vi "Slog1.vi"(2 "z":dbl[](array[numeric]), 3 "T":dbl[](array[numeric])) -> (0 "dY":dbl[](array[numeric]), 1 "Y":dbl[](array[numeric]))   [LabVIEW 2022 SP3]
uses:
  <vilib>/express/express arith-compare/Formula/XNode/ExpressFormulaBlockNode.xnode
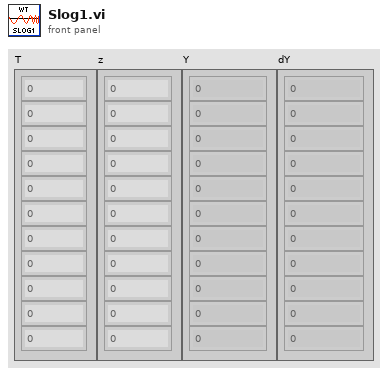
[diagram p1: front panel]
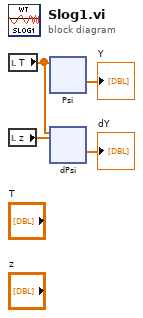
[diagram p0: block diagram]
diagram:
  n1 = local read "T"() -> (w3:dbl[])
  n2 = local read "z"() -> (w2:dbl[])
  n3 = xnode "Psi"("t"=w3) -> ("Result"=→"Y":dbl[])  [unwired: 1 in, 1 out]
  n4 = xnode "dPsi"("t"=w3, "a"=w2) -> ("Result"=→"dY":dbl[])  [unwired: 1 in, 1 out]
